vi "Data to List.vi"(0 "Data String In":string, 11 "error in":errorcluster) -> (4 "Data List Out":refnum<k24>, 15 "error out":errorcluster)   [LabVIEW 2014, in "GEA2_Toolkit.lvlib"]
uses:
  library/GEA2_Toolkit.lvlib
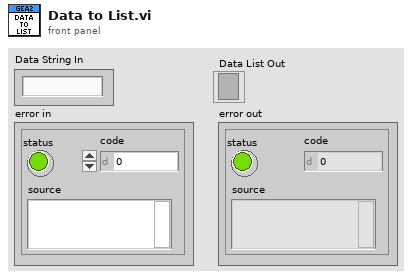
[diagram p1: front panel]
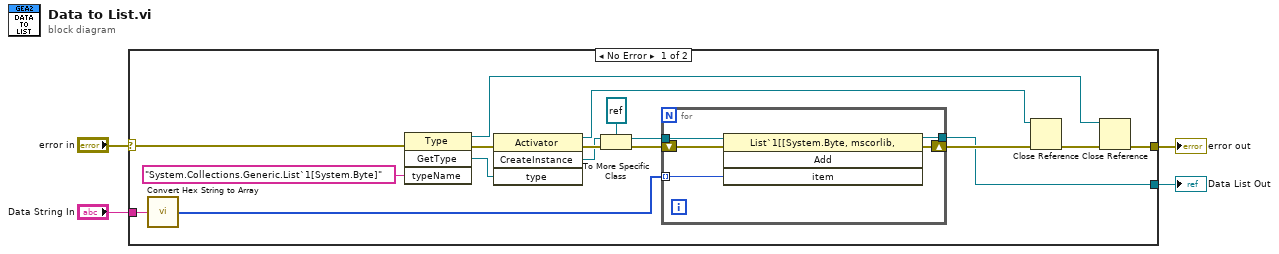
[diagram p0: block diagram]
diagram:
  n1 = case shown="No Error" "error in" {
    selector: "error in" -> [w5 w27]
    tunnel: [w10 _] -> w4
    tunnel: [w9 w27] -> w3
    tunnel: "Data String In" -> [w8 _]
    frame No Error {
      n2 = call "Convert Hex String to Array.vi"("Hex String In"=w8) -> ("Hex Array Out"=w13:u8[])  [unwired: 13 in, 1 out]
      n3 = invoke class="Type" method="GetType"(error in=w5, "typeName"="System.Collections.Generic.List`1[System.Byte]") -> (reference out=w6:refnum<k24>, error out=w20:errorcluster, "GetType"=w21:refnum<k24>)  [unwired: 2 in, 1 out]
      n4 = invoke class="Activator" method="CreateInstance"(error in=w20, "type"=w21) -> (reference out=w7:refnum<k24>, error out=w18:errorcluster, "CreateInstance"=w15:refnum<k24>)  [unwired: 2 in, 1 out]
      n5 = To More Specific Class(target class=refnum<k24> refnum ("reference"), reference=w15, error in=w18) -> (specific class reference=w17:refnum<k24>, error out=w16:errorcluster)
      n6 = for {
        tunnel: [w26] -> w10
        tunnel: w13 -> [w25] mode=indexing
        shift-right: [w24] -> w11
        shift-left: w16 -> [w23]
        tunnel: w17 -> [w22]
        n7 = invoke class="List`1[[System.Byte, mscorlib, " method="Add"(reference=w22, error in=w23, "item"=w25) -> (reference out=w26:refnum<k24>, error out=w24:errorcluster)  [unwired: 1 in, 2 out]
      }
      n8 = Close Reference(reference=w7, error in (no error)=w11) -> (error out=w12:errorcluster)
      n9 = Close Reference(reference=w6, error in (no error)=w12) -> (error out=w9:errorcluster)
    }
    frame Error {
    }
  }
  "Data List Out" <- w4
  "error out" <- w3
